vi "Prod - Read Settings.vi"(8 "Error In":errorcluster, 11 "Prod Data In":T2={"Queue_Producer"=refnum, "Queue_Consumer"=refnum, "To_GUI-Error_message"=refnum, "Rx-Data"=[], "Tx-Data"=[], "Console log"="", "Communication Settings"={"Tx Protocol"=enum."Not Active", "Rx Protocol"=enum."Serial", "Serial"={"Tx Port"="", "Rx Port"="", "Baud rate"=0, "Parity"=enum."Space", "Data bits"=0, "Stop bits"=0, "Flow control"=enum."None", "Tx Resource"="", "Rx Resource"=""}, "MIDI Device"={"Input uDevice ID"=0, "Output uDevice ID"=0, "hmidiout Handle"=0, "hmidiin Handle"=0}, "Bluetooth"={"Dummy"=""}, "USB"={"Dummy"=""}}, "MIDI-Messages"=[], "Queue_Session"=refnum, "To_GUI-Pre-Session"=refnum, "To_GUI-Producer"=refnum, "Tx Info"={"Datatype"=[], "Bytesize"=[], "Strings"=[], "ByteSum"=0}, "Payload"=variant, "Timout-Time[ms]"=0, "To_GUI-Session"=refnum, "CPU(ms)"=0}) -> (0 "Error Out":errorcluster, 3 "Prod Data Out":T2={"Queue_Producer"=refnum, "Queue_Consumer"=refnum, "To_GUI-Error_message"=refnum, "Rx-Data"=[], "Tx-Data"=[], "Console log"="", "Communication Settings"={"Tx Protocol"=enum."Not Active", "Rx Protocol"=enum."Serial", "Serial"={"Tx Port"="", "Rx Port"="", "Baud rate"=0, "Parity"=enum."Space", "Data bits"=0, "Stop bits"=0, "Flow control"=enum."None", "Tx Resource"="", "Rx Resource"=""}, "MIDI Device"={"Input uDevice ID"=0, "Output uDevice ID"=0, "hmidiout Handle"=0, "hmidiin Handle"=0}, "Bluetooth"={"Dummy"=""}, "USB"={"Dummy"=""}}, "MIDI-Messages"=[], "Queue_Session"=refnum, "To_GUI-Pre-Session"=refnum, "To_GUI-Producer"=refnum, "Tx Info"={"Datatype"=[], "Bytesize"=[], "Strings"=[], "ByteSum"=0}, "Payload"=variant, "Timout-Time[ms]"=0, "To_GUI-Session"=refnum, "CPU(ms)"=0})   [LabVIEW 2019]
doc: "Reads new settings for producer."
uses:
  Controls/Producer-Data.ctl
  Common/Controls/Application_Message.ctl
  Common/Controls/Application_State.ctl
  Common/Controls/Communication_Settings.ctl
  Common/Controls/Communication_Protocols.ctl
  MIDI/Controls/MIDI-Message_Array.ctl
  MIDI/Controls/MIDI-Message_Cluster.ctl
  MIDI/Controls/Meta_Commands.ctl
  Controls/Prod - Tx_Info.ctl
panel:
  in  "Control Tab":T1(tab)
  out "Console Log":string
  out "VI-filename":string
  out "VI Path":path
  out "Code Size":u32
  out "Revision Number":u32
  in  "Tool Bar:Visible":bool
  in  "Execution:Show Front Panel On Call":bool
  out "VI-Name":string
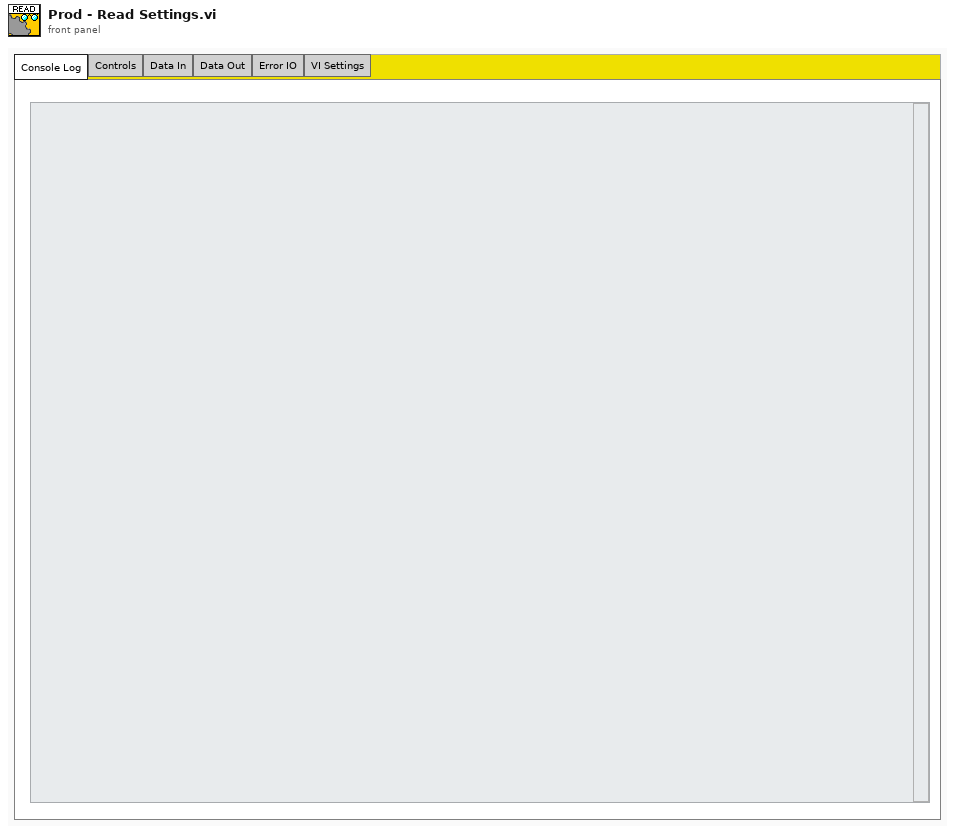
[diagram p1: front panel]
types:
  T1 = enum32{"Console Log", "Controls", "Data In", "Data Out", "Error IO", "VI Settings"}
  T2 = typedef "Producer-Data.ctl" = cluster{"Queue_Producer":refnum<queue>, "Queue_Consumer":refnum<queue>, "To_GUI-Error_message":refnum<user-event>, "Rx-Data":i8[], "Tx-Data":i8[], "Console log":string, "Communication Settings":T3, "MIDI-Messages":T5, "Queue_Session":refnum<queue>, "To_GUI-Pre-Session":refnum<user-event>, "To_GUI-Producer":refnum<user-event>, "Tx Info":T8, "Payload":variant, "Timout-Time[ms]":i32, "To_GUI-Session":refnum<user-event>, "CPU(ms)":u32}
  T3 = typedef "Communication_Settings.ctl" = cluster{"Tx Protocol":T4, "Rx Protocol":T4, "Serial":cluster{"Tx Port":refnum<visa-resource-name>, "Rx Port":refnum<visa-resource-name>, "Baud rate":i32, "Parity":enum16{"None", "Odd", "Even", "Mark", "Space"}, "Data bits":i32, "Stop bits":i32, "Flow control":enum16{"None", "XON/XOFF", "RTS/CTS", "XON/XOFF & RTS/CTS", "DTR/DSR", "XON/XOFF & DTR/DSR"}, "Tx Resource":refnum<visa-resource-name>, "Rx Resource":refnum<visa-resource-name>}, "MIDI Device":cluster{"Input uDevice ID":u32, "Output uDevice ID":u32, "hmidiout Handle":i32, "hmidiin Handle":i32}, "Bluetooth":cluster{"Dummy":string}, "USB":cluster{"Dummy":string}}
  T4 = typedef "Communication_Protocols.ctl" = enum16{"Serial", "Bluetooth", "USB-MIDI", "MIDI (Audio Device)", "Not Active"}
  T5 = typedef "MIDI-Message_Array.ctl" = T6[]
  T6 = typedef "MIDI-Message_Cluster.ctl" = cluster{"Message Name":string, "Meta value":i32, "Datastring":string, "Datatype":T7}
  T7 = typedef "Meta_Commands.ctl" = enum16{"No Data", "Pause", "Loop", "Wait for Rx", "Delay", "Break", "MIDI"}
  T8 = typedef "Prod - Tx_Info.ctl" = cluster{"Datatype":T7[], "Bytesize":i32[], "Strings":string[], "ByteSum":i32}
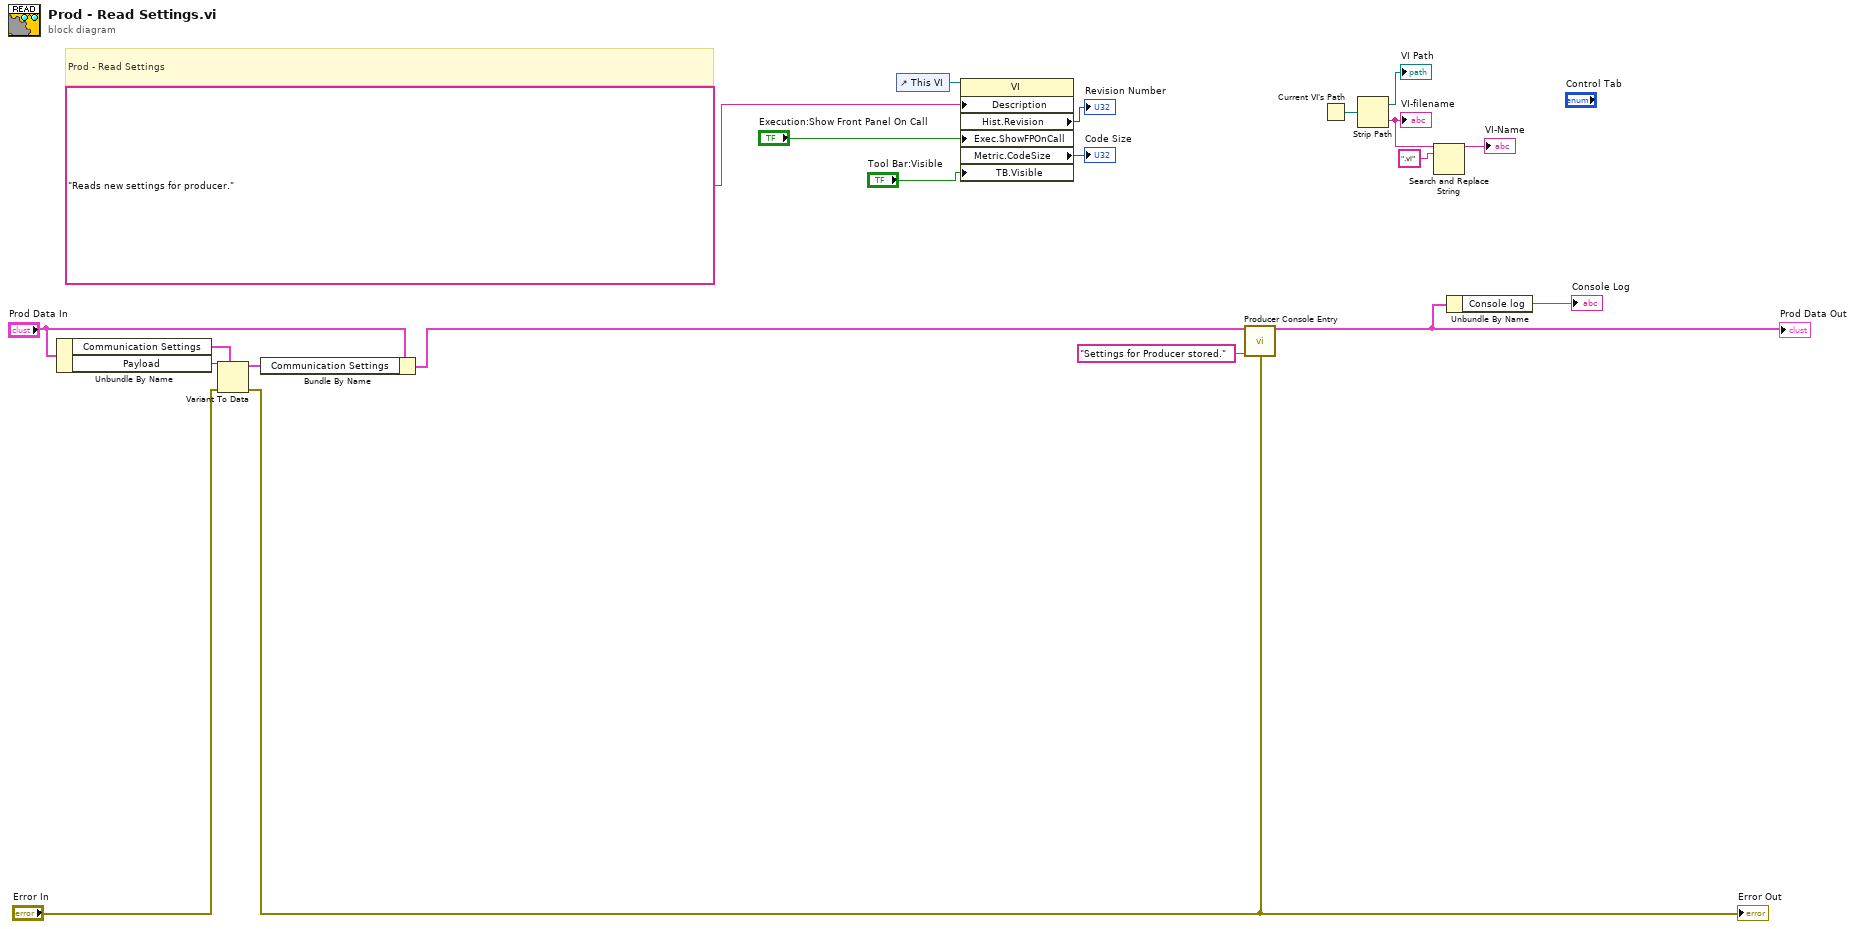
[diagram p0: block diagram]
diagram:
  # "Prod - Read Settings"
  n1 = Unbundle By Name("Prod Data In") -> ("Communication Settings"=w9:T3, "Payload"=w8:variant)
  n2 = Variant To Data(error in="Error In", type=w9, Variant=w8) -> (data=w10:T3, error out=w6:errorcluster)
  "Error Out" <- w6
  n3 = Bundle By Name(cluster="Prod Data In", "Communication Settings"=w10) -> (w1:T2)
  n4 = control-ref of="This VI"() -> (w15:refnum<vi>)
  n5 = property class="VI"(reference=w15, "Description"="Reads new settings for producer.", "Exec.ShowFPOnCall"="Execution:Show Front Panel On Call", "TB.Visible"="Tool Bar:Visible") -> ("Hist.Revision"=→"Revision Number":u32, "Metric.CodeSize"=→"Code Size":u32)  [unwired: 1 in, 2 out]
  n6 = call "Producer Console Entry.vi"("Prod-Data In"=w1, "Console Entry"="Settings for Producer stored.", "Error In"=w6) -> ("Prod-Data Out"=w3:T2)  [unwired: 12 in]
  "Prod Data Out" <- w3
  n7 = Current VI's Path() -> (path=w21:path)
  n8 = Strip Path(path=w21) -> (stripped path=→"VI Path":path, name=w12:string)
  "VI-filename" <- w12
  n9 = Search and Replace String(input string=w12, search string=".vi") -> (result string=→"VI-Name":string)  [unwired: 6 in, 3 out]
  n10 = Unbundle By Name(w3) -> ("Console log"=→"Console Log":string)
